vi "ActualBarcodeReader3.vi"(11 "NXT/EV3":T1) -> (0 "O HPE":i32, 1 "Blue Small":i32, 2 "Red Small":i32, 3 "White Small":i32, 4 "Steel":i32, 5 "NXT/EV3 2":T1, 8 "White Large":i32, 9 "Red Large":i32, 10 "Blue Large":i32)   [LabVIEW 2016]
uses:
  <vilib>/NXT/Subs/LVHSConnector.ctl
  <vilib>/NXT/LegoClasses/BrickReference/BrickReference.lvclass
  <vilib>/NXT/Subs/ColorSensorColors.ctl
  <vilib>/NXT/Block Support/NXT_InputPort.ctl
  <vilib>/NXT/Block Support/NXT_OutputPort.ctl
  <vilib>/NXT/NXTIO Xnodes/NXTIONodeSubVIs/NXTMoveMotors.vi
  <vilib>/NXT/Dual Mode Library/Waits/Wait_EV3_Color_Color.vi
  <vilib>/NXT/NXTIO Xnodes/NXTIONodeSubVIs/NXTStopMotors.vi
  <vilib>/NXT/NXTIO Xnodes/NXTIONodeSubVIs/NXTMotorRunDistance.vi
  <vilib>/NXT/Dual Mode Library/Waits/Wait_Num.vi
  <vilib>/NXT/NXTIO Xnodes/AddressXNode/NXTIOAddress.xnode
  <vilib>/NXT/NXTIO Xnodes/NXTIOXNode/NXTIO.xnode
panel:
  out "Type 2 Count":string
  out "Type 1 Count":string
  out "Material":string
  out "Type 1 & Type 2":i32
  out "Material":i32
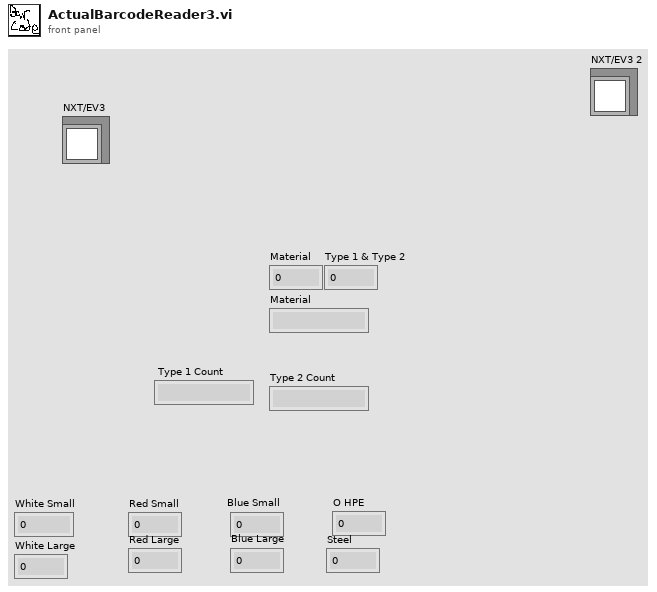
[diagram p1: front panel]
types:
  T1 = typedef "LVHSConnector.ctl" = refnum<class "BrickReference.lvclass">
  T2 = typedef "ColorSensorColors.ctl" = enum16{"No Color", "Black", "Blue", "Green", "Yellow", "Red", "White", "Brown"}
  T3 = typedef "NXT_InputPort.ctl" = u32
  T4 = typedef "NXT_OutputPort.ctl" = u8
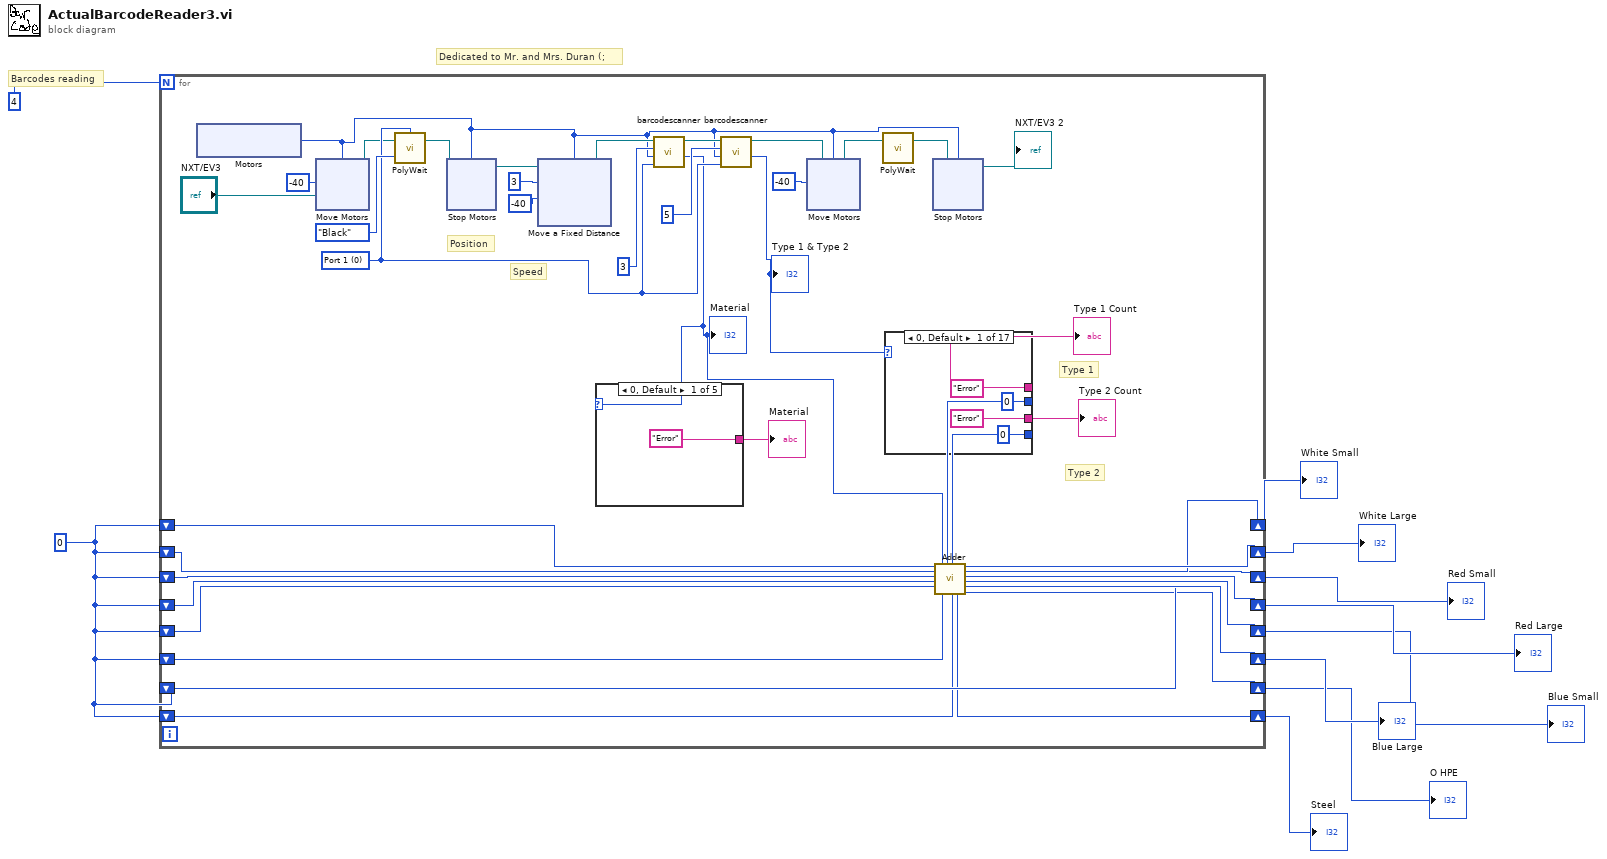
[diagram p0: block diagram]
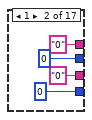
[diagram p2: hidden frame]
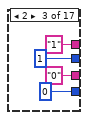
[diagram p3: hidden frame]
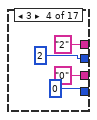
[diagram p4: hidden frame]
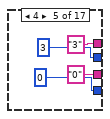
[diagram p5: hidden frame]
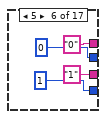
[diagram p6: hidden frame]
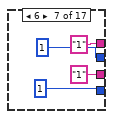
[diagram p7: hidden frame]
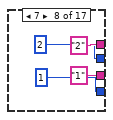
[diagram p8: hidden frame]
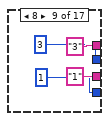
[diagram p9: hidden frame]
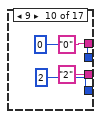
[diagram p10: hidden frame]
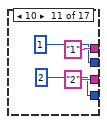
[diagram p11: hidden frame]
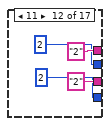
[diagram p12: hidden frame]
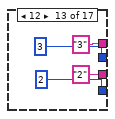
[diagram p13: hidden frame]
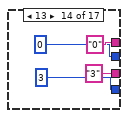
[diagram p14: hidden frame]
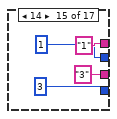
[diagram p15: hidden frame]
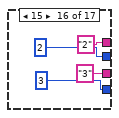
[diagram p16: hidden frame]
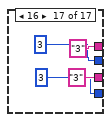
[diagram p17: hidden frame]
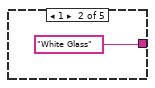
[diagram p18: hidden frame]
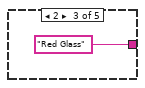
[diagram p19: hidden frame]
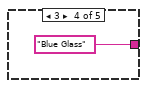
[diagram p20: hidden frame]
diagram:
  w9 = 0
  # "Dedicated to Mr. and Mrs. Duran (;"
  # "Barcodes reading"
  n1 = for {
    N: 4 -> [_]
    shift-right: [w27] -> w5
    shift-left: w9 -> [w28]
    shift-right: [w29] -> w6
    shift-left: w9 -> [w30]
    shift-right: [w23] -> w3
    shift-left: w9 -> [w25]
    shift-right: [w21] -> w2
    shift-left: w9 -> [w22]
    shift-right: [w31] -> w8
    shift-left: w9 -> [w34]
    shift-right: [w24] -> w4
    shift-left: w9 -> [w26]
    shift-right: [w19] -> w1
    shift-left: w9 -> [w20]
    shift-right: [w32] -> w7
    shift-left: w9 -> [w33]
    w46 = T3 0 items=["Port 1", "Port 2", "Port 3", "Port 4"] ("Port (Port 1)")
    # "Type 2"
    # "Type 1"
    # "Position"
    # "Speed"
    n2 = xnode "Motors"() -> ("Motor"=w13:T4)
    n3 = xnode "Move Motors"("Power/Speed 1"=i8 -40, "Motors"=w13, "NXT/EV3"="NXT/EV3") -> ("NXT/EV3"=w17:T1)
    n4 = call-poly <vilib>:"PolyWait.vi"("Color (Red)"=ColorSensorColors."Black", "NXT/EV3"=w17, "Port (Port 1)"=w46) -> ("NXT/EV3"=w16:T1)  [unwired: 1 in]
    n5 = xnode "Stop Motors"("Motors"=w13, "NXT/EV3"=w16) -> ("NXT/EV3"=w15:T1)
    n6 = xnode "Move a Fixed Distance"("Speed 1"=-40, "Distance 1"=3, "Motors"=w13, "NXT/EV3"=w15) -> ("NXT/EV3"=w14:T1)
    n7 = call "barcodescanner.vi"("Color Sensor Port"=w46, "Motors"=w13, "digits"=3, "NXT/EV3"=w14) -> ("decimal conversiom"=w38:i32, "NXT/EV3 2"=w48:T1)  [unwired: 6 in]
    "Material" <- w38
    n8 = case shown="0, Default" w38 {
      tunnel: ["Error" "White Glass" "Red Glass" "Blue Glass" "Steel/HDPE"] -> w35
      frame 0, Default {
      }
      frame 1 {
      }
      frame 2 {
      }
      frame 3 {
      }
      frame 4 {
      }
    }
    "Material" <- w35
    n9 = call "barcodescanner.vi"("Color Sensor Port"=w46, "Motors"=w13, "digits"=5, "NXT/EV3"=w48) -> ("decimal conversiom"=w40:i32, "NXT/EV3 2"=w45:T1)  [unwired: 6 in]
    "Type 1 & Type 2" <- w40
    n10 = xnode "Move Motors"("Power/Speed 1"=i8 -40, "Motors"=w13, "NXT/EV3"=w45) -> ("NXT/EV3"=w43:T1)
    n11 = call-poly <vilib>:"PolyWait.vi"("NXT/EV3"=w43) -> ("NXT/EV3"=w42:T1)  [unwired: 3 in]
    n12 = case shown="0, Default" w40 {
      tunnel: ["Error" "0" "1" "2" "3" "0" "1" "2" "3" "0" "1" "2" "3" "0" "1" "2" "3"] -> w41
      tunnel: ["Error" "0" "0" "0" "0" "1" "1" "1" "1" "2" "2" "2" "2" "3" "3" "3" "3"] -> w39
      tunnel: [0 0 1 2 3 0 1 2 3 0 1 2 3 0 1 2 3] -> w37
      tunnel: [0 0 0 0 0 1 1 1 1 2 2 2 2 3 3 3 3] -> w36
      frame 0, Default {
      }
      frame 1 {
      }
      frame 2 {
      }
      frame 3 {
      }
      frame 4 {
      }
      frame 5 {
      }
      frame 6 {
      }
      frame 7 {
      }
      frame 8 {
      }
      frame 9 {
      }
      frame 10 {
      }
      frame 11 {
      }
      frame 12 {
      }
      frame 13 {
      }
      frame 14 {
      }
      frame 15 {
      }
      frame 16 {
      }
    }
    "Type 1 Count" <- w41
    "Type 2 Count" <- w39
    n13 = xnode "Stop Motors"("Motors"=w13, "NXT/EV3"=w42) -> ("NXT/EV3"=→"NXT/EV3 2":T1)
    n14 = call "Adder.vi"("I White Small"=w34, "I White Large"=w33, "I Red Small"=w30, "I Red Large"=w28, "I Blue Small"=w26, "Material"=w38, "I Blue Large"=w25, "Type 1"=w37, "I HPDE"=w22, "Type 2"=w36, "I Steel"=w20) -> ("O White Small"=w31:i32, "O Steel"=w19:i32, "O White Large"=w32:i32, "O Red Small"=w29:i32, "O Red Large"=w27:i32, "O Blue Small"=w24:i32, "O Blue Large"=w23:i32, "O HPDE"=w21:i32)  [unwired: 1 in]
  }
  "White Small" <- w8
  "White Large" <- w7
  "Red Small" <- w6
  "Red Large" <- w5
  "Blue Small" <- w4
  "Blue Large" <- w3
  "O HPE" <- w2
  "Steel" <- w1
